vi "Driver_selection.vi"(4 "error in (no error) 2":errorcluster, 6 "JoystickDevRef 2":T1, 8 "error in (no error) 1":errorcluster, 9 "JoystickDevRef 1":T1, 10 "error in (no error) 0":errorcluster, 11 "JoystickDevRef 0":T1) -> ()   [LabVIEW 2017]
uses:
  <vilib>/Rock Robotics/WPI/Joystick/WPI_JoystickDevRef.ctl
  <vilib>/Rock Robotics/WPI/Joystick/WPI_JoystickDeviceEnum.ctl
  <vilib>/Rock Robotics/Network Tables/SD Write Boolean Array.vi
  <vilib>/Rock Robotics/WPI/Utilities/WPI_GetSetVariantRefNum.vi
  <vilib>/Rock Robotics/WPI/RobotDrive/WPI_RobotDriveMecanumDrive_Cartesian.vi
  <vilib>/Rock Robotics/Network Tables/SD Write Numeric Array.vi
  <vilib>/Rock Robotics/Network Tables/NT Read Boolean.vi
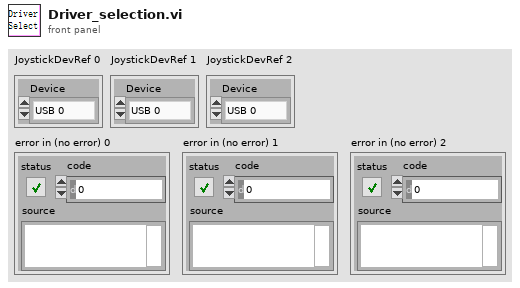
[diagram p1: front panel]
types:
  T1 = typedef "WPI_JoystickDevRef.ctl" = cluster{"Device":T2}
  T2 = typedef "WPI_JoystickDeviceEnum.ctl" = enum16{"USB 0", "USB 1", "USB 2", "USB 3", "USB 4", "USB 5"}
  T3 = typedef "WPI_MotorControlDeviceRef.ctl" = cluster{"DeviceStatus":errorcluster, "Type":T4, "PWM":cluster{"PWM Channel":T5, "DeadBand":T6}, "CAN":cluster{"Device Number":u8, "SetOutput VI Ref":variant, "GetOutput VI Ref":variant, "Enable VI Ref":variant, "Disable VI Ref":variant, "Data":variant}, "Invert":bool, "DIO PWM":cluster{"PWM \"Enable\" Channel":T5, "DIOChannel":T7, "PWM Rate":dbl}}
  T4 = typedef "WPI_MotorControlType.ctl" = enum16{"PWM", "CAN", "DIO PWM"}
  T5 = typedef "FPGA_DIOPWMChannel.ctl" = enum8{"PWM 0", "PWM 1", "PWM 2", "PWM 3", "PWM 4", "PWM 5", "PWM 6", "PWM 7", "PWM 8", "PWM 9", "PWM MXP 0", "PWM MXP 1", "PWM MXP 2", "PWM MXP 3", "PWM MXP 4", "PWM MXP 5", "PWM MXP 6", "PWM MXP 7", "PWM MXP 8", "PWM MXP 9", "Invalid"}
  T6 = typedef "WPI_PWMDeadband.ctl" = cluster{"Name":string, "maxPositivePwm":i32, "minPositivePwm":i32, "centerPwm":i32, "maxNegativePwm":i32, "minNegativePwm":i32, "angularRange":u16}
  T7 = typedef "FPGA_DIOChannel.ctl" = enum8{"DIO 0", "DIO 1", "DIO 2", "DIO 3", "DIO 4", "DIO 5", "DIO 6", "DIO 7", "DIO 8", "DIO 9", "DIO MXP 0", "DIO MXP 1", "DIO MXP 2", "DIO MXP 3", "DIO MXP 4", "DIO MXP 5", "DIO MXP 6", "DIO MXP 7", "DIO MXP 8", "DIO MXP 9", "DIO MXP 10", "DIO MXP 11", "DIO MXP 12", "DIO MXP 13", "DIO MXP 14", "DIO MXP 15", "SPI Port CS1", "SPI Port CS2", "SPI Port CS3", "SPI Port MISO", "SPI Port MOSI", "Invalid"}
  T8 = typedef "WPI_RobotDriveDevRef.ctl" = cluster{"DevStatus":errorcluster, "Motors[]":T3[], "Square Inputs":bool, "Max Output":dbl}
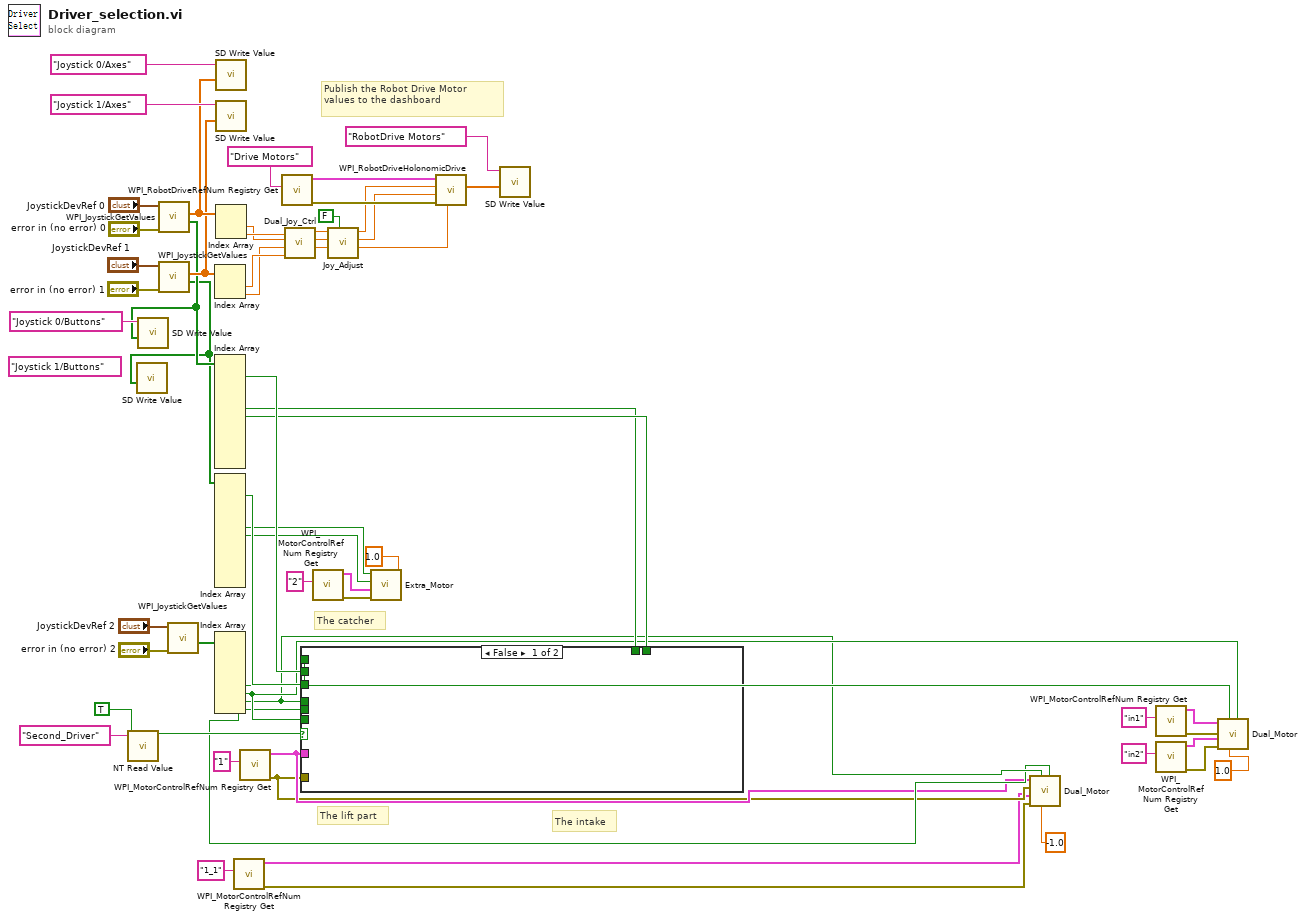
[diagram p0: block diagram]
diagram:
  (unwired) "Joystick 1/Buttons" ("Name")
  # "The lift part"
  # "The intake"
  # "The catcher"
  # "Publish the Robot Drive Motor\nvalues to the dashboard"
  n1 = call-poly <vilib>:"NT Read Value.vi"("Default Value"=TRUE, "Name"="Second_Driver") -> ("Boolean"=w33:bool)  [unwired: 8 in, 1 out]
  n2 = call <vilib>:"WPI_JoystickGetValues.vi"("error in (no error)"="error in (no error) 0", "JoystickDevRef"="JoystickDevRef 0") -> ("Buttons"=w30:bool[], "Axes"=w37:dbl[])  [unwired: 5 in, 3 out]
  n3 = call-poly <vilib>:"SD Write Value.vi"("Boolean Array"=w30, "Name"="Joystick 0/Buttons") -> ()  [unwired: 8 in, 2 out]
  n4 = call <vilib>:"WPI_JoystickGetValues.vi"("error in (no error)"="error in (no error) 1", "JoystickDevRef"="JoystickDevRef 1") -> ("Buttons"=w29:bool[], "Axes"=w36:dbl[])  [unwired: 5 in, 3 out]
  n5 = call-poly <vilib>:"SD Write Value.vi"("Boolean Array"=w29) -> ()  [unwired: 9 in, 2 out]
  n6 = call <vilib>:"WPI_JoystickGetValues.vi"("error in (no error)"="error in (no error) 2", "JoystickDevRef"="JoystickDevRef 2") -> ("Buttons"=w32:bool[])  [unwired: 5 in, 4 out]
  n7 = Index Array(array=w36) -> (element #1=w53:dbl, element #2=w52:dbl)  [unwired: 2 in]
  n8 = Index Array(array=w30) -> (element #1=w28:bool, element #5=w19:bool, element #6=w20:bool)  [unwired: 12 in, 9 out]
  n9 = Index Array(array=w29) -> (element #1=w27:bool, element #5=w22:bool, element #6=w21:bool)  [unwired: 12 in, 9 out]
  n10 = Index Array(array=w32) -> (element #5=w18:bool, element #6=w17:bool, element #7=w7:bool, element #8=w6:bool)  [unwired: 8 in, 4 out]
  n11 = call-poly <vilib>:"SD Write Value.vi"("Numeric Array"=w37, "Name"="Joystick 0/Axes") -> ()  [unwired: 8 in, 2 out]
  n12 = call-poly <vilib>:"SD Write Value.vi"("Numeric Array"=w36, "Name"="Joystick 1/Axes") -> ()  [unwired: 8 in, 2 out]
  n13 = Index Array(array=w37) -> (element #1=w54:dbl, element #2=w55:dbl)  [unwired: 2 in]
  n14 = call <vilib>:"WPI_MotorControlRefNum Registry Get.vi"("refnum name"="1_1") -> ("error out"=w2:errorcluster, "MotorControlDevRef"=w3:T3)  [unwired: 9 in]
  n15 = call <vilib>:"WPI_MotorControlRefNum Registry Get.vi"("refnum name"="1") -> ("error out"=w4:errorcluster, "MotorControlDevRef"=w5:T3)  [unwired: 9 in]
  n16 = call <vilib>:"WPI_RobotDriveRefNum Registry Get.vi"("refnum name"="Drive Motors") -> ("error out"=w43:errorcluster, "RobotDriveDevRef"=w46:T8)  [unwired: 1 in, 8 out]
  n17 = call "Dual_Joy_Ctrl.vi"("Joy1_0(X)"=w53, "Joy1_1(Y)"=w52, "Joy0_0(X)"=w54, "Joy0_1(Y)"=w55) -> ("Z"=w49:dbl, "Y"=w50:dbl, "X"=w51:dbl)  [unwired: 5 in]
  n18 = case shown="False" w33 {
    tunnel: w7 -> [_ _]
    tunnel: w6 -> [_ _]
    tunnel: w5 -> [_ _]
    tunnel: w4 -> [_ _]
    tunnel: w28 -> [_ _]
    tunnel: w27 -> [_ _]
    tunnel: w20 -> [_ _]
    tunnel: w19 -> [_ _]
    tunnel: w18 -> [_ _]
    tunnel: w17 -> [_ _]
    frame False {
    }
    frame True {
    }
  }
  n19 = call <vilib>:"WPI_MotorControlRefNum Registry Get.vi"("refnum name"="2") -> ("error out"=w25:errorcluster, "MotorControlDevRef"=w24:T3)  [unwired: 9 in]
  n20 = call "Joy_Adjust.vi"("Rotation Special Adjust?"=FALSE, "Rotation"=w49, "Y"=w50, "X"=w51) -> ("Rotation'"=w40:dbl, "Y'"=w41:dbl, "X'"=w42:dbl)  [unwired: 5 in]
  n21 = call "Extra_Motor.vi"("Speed"=1.0, "error in (no error)"=w25, "MotorControlDevRef"=w24, "Backward"=w21, "Forward"=w22) -> ()  [unwired: 6 in]
  n22 = call-poly <vilib>:"WPI_RobotDriveHolonomicDrive.vi"("Rotation"=w40, "error in (no error)"=w43, "Y"=w41, "X"=w42, "RobotDriveDevRef"=w46) -> ("Motor Values"=w44:dbl[])  [unwired: 4 in, 2 out]
  n23 = call-poly <vilib>:"SD Write Value.vi"("Numeric Array"=w44, "Name"="RobotDrive Motors") -> ()  [unwired: 8 in, 2 out]
  n24 = call "Dual_Motor.vi"("Backward"=w6, "Speed"=-1.0, "Forward"=w7, "error in (no error) 2"=w2, "MotorControlDevRef 2"=w3, "error in (no error)"=w4, "MotorControlDevRef"=w5) -> ()  [unwired: 5 in]
  n25 = call <vilib>:"WPI_MotorControlRefNum Registry Get.vi"("refnum name"="in1") -> ("error out"=w14:errorcluster, "MotorControlDevRef"=w15:T3)  [unwired: 9 in]
  n26 = call <vilib>:"WPI_MotorControlRefNum Registry Get.vi"("refnum name"="in2") -> ("error out"=w12:errorcluster, "MotorControlDevRef"=w13:T3)  [unwired: 9 in]
  n27 = call "Dual_Motor.vi"("Backward"=w17, "Speed"=1.0, "Forward"=w18, "error in (no error) 2"=w12, "MotorControlDevRef 2"=w13, "error in (no error)"=w14, "MotorControlDevRef"=w15) -> ()  [unwired: 5 in]
